vi "generateInitialTriggerTimes.vi"() -> (1 "Trigger message":T2)   [LabVIEW 2017]
doc: "Generate dummy start times for the trigger loop so nothing weird happens before the first trigger."
uses:
  Trigger message.ctl
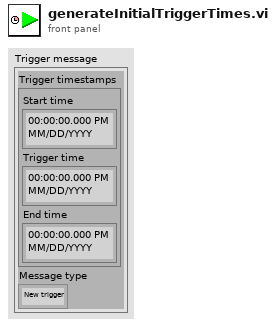
[diagram p1: front panel]
types:
  T1 = typedef "Trigger message.ctl" = enum16{"New trigger", "Updated trigger"}
  T2 = cluster{"Trigger timestamps":cluster{"Start time":timestamp, "Trigger time":timestamp, "End time":timestamp}, "Message type":T1}
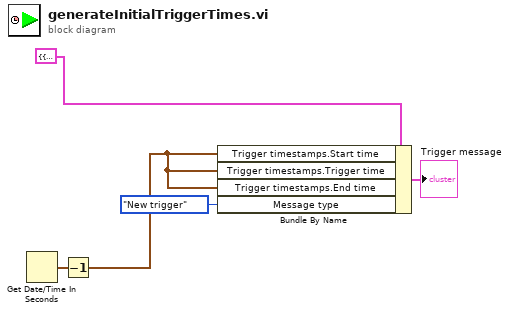
[diagram p0: block diagram]
diagram:
  n1 = Get Date/Time In Seconds() -> (seconds since 1Jan1904=w5:timestamp)
  n2 = Decrement(x=w5) -> (x-1=w3:timestamp)
  n3 = Bundle By Name(cluster=T2 {"Trigger timestamps"={"Start time"=timestamp(0 s since 1904-01-01), "Trigger time"=timestamp(0 s since 1904-01-01), "End time"=timestamp(0 s since 1904-01-01)}, "Message type"=enum."New trigger"} ("Trigger message"), "Trigger timestamps.Start time"=w3, "Trigger timestamps.Trigger time"=w3, "Trigger timestamps.End time"=w3, "Message type"=Trigger_message."New trigger") -> (→"Trigger message":T2)
